vi "TxData_Organization_EVM_EIRP_Max.vi"() -> ()   [LabVIEW 2023, in "ParsingData.lvlib"]
uses:
  <vilib>/Utility/file.llb/Read Delimited Spreadsheet (string).vi
  <vilib>/Utility/file.llb/Read Delimited Spreadsheet (DBL).vi
  ParsingData.lvlib
panel:
  out "Best EVM":T1(array[cluster])
  in  "EIRP_res":dbl=10.0
  in  "EIRP_Max":dbl
  in  "EIRP_Min":dbl=-60.0
  in  "CalPower ¸ÉÀv":dbl=70.0 format="%#_13g"
  in  "Input power_res":dbl=10.0
  in  "Input power_up":dbl
  in  "Input power_low":dbl=-60.0
  in  "File Path":path
  out "Max EVM : Mode             Polarity                     UD att                BFIC COM att           BFIC ele att                SG Power                      EIRP                           EVM":string[](array[string])
  out "EVM to EIRP":cluster{dbl[], "all rows":dbl[]}[](graph)
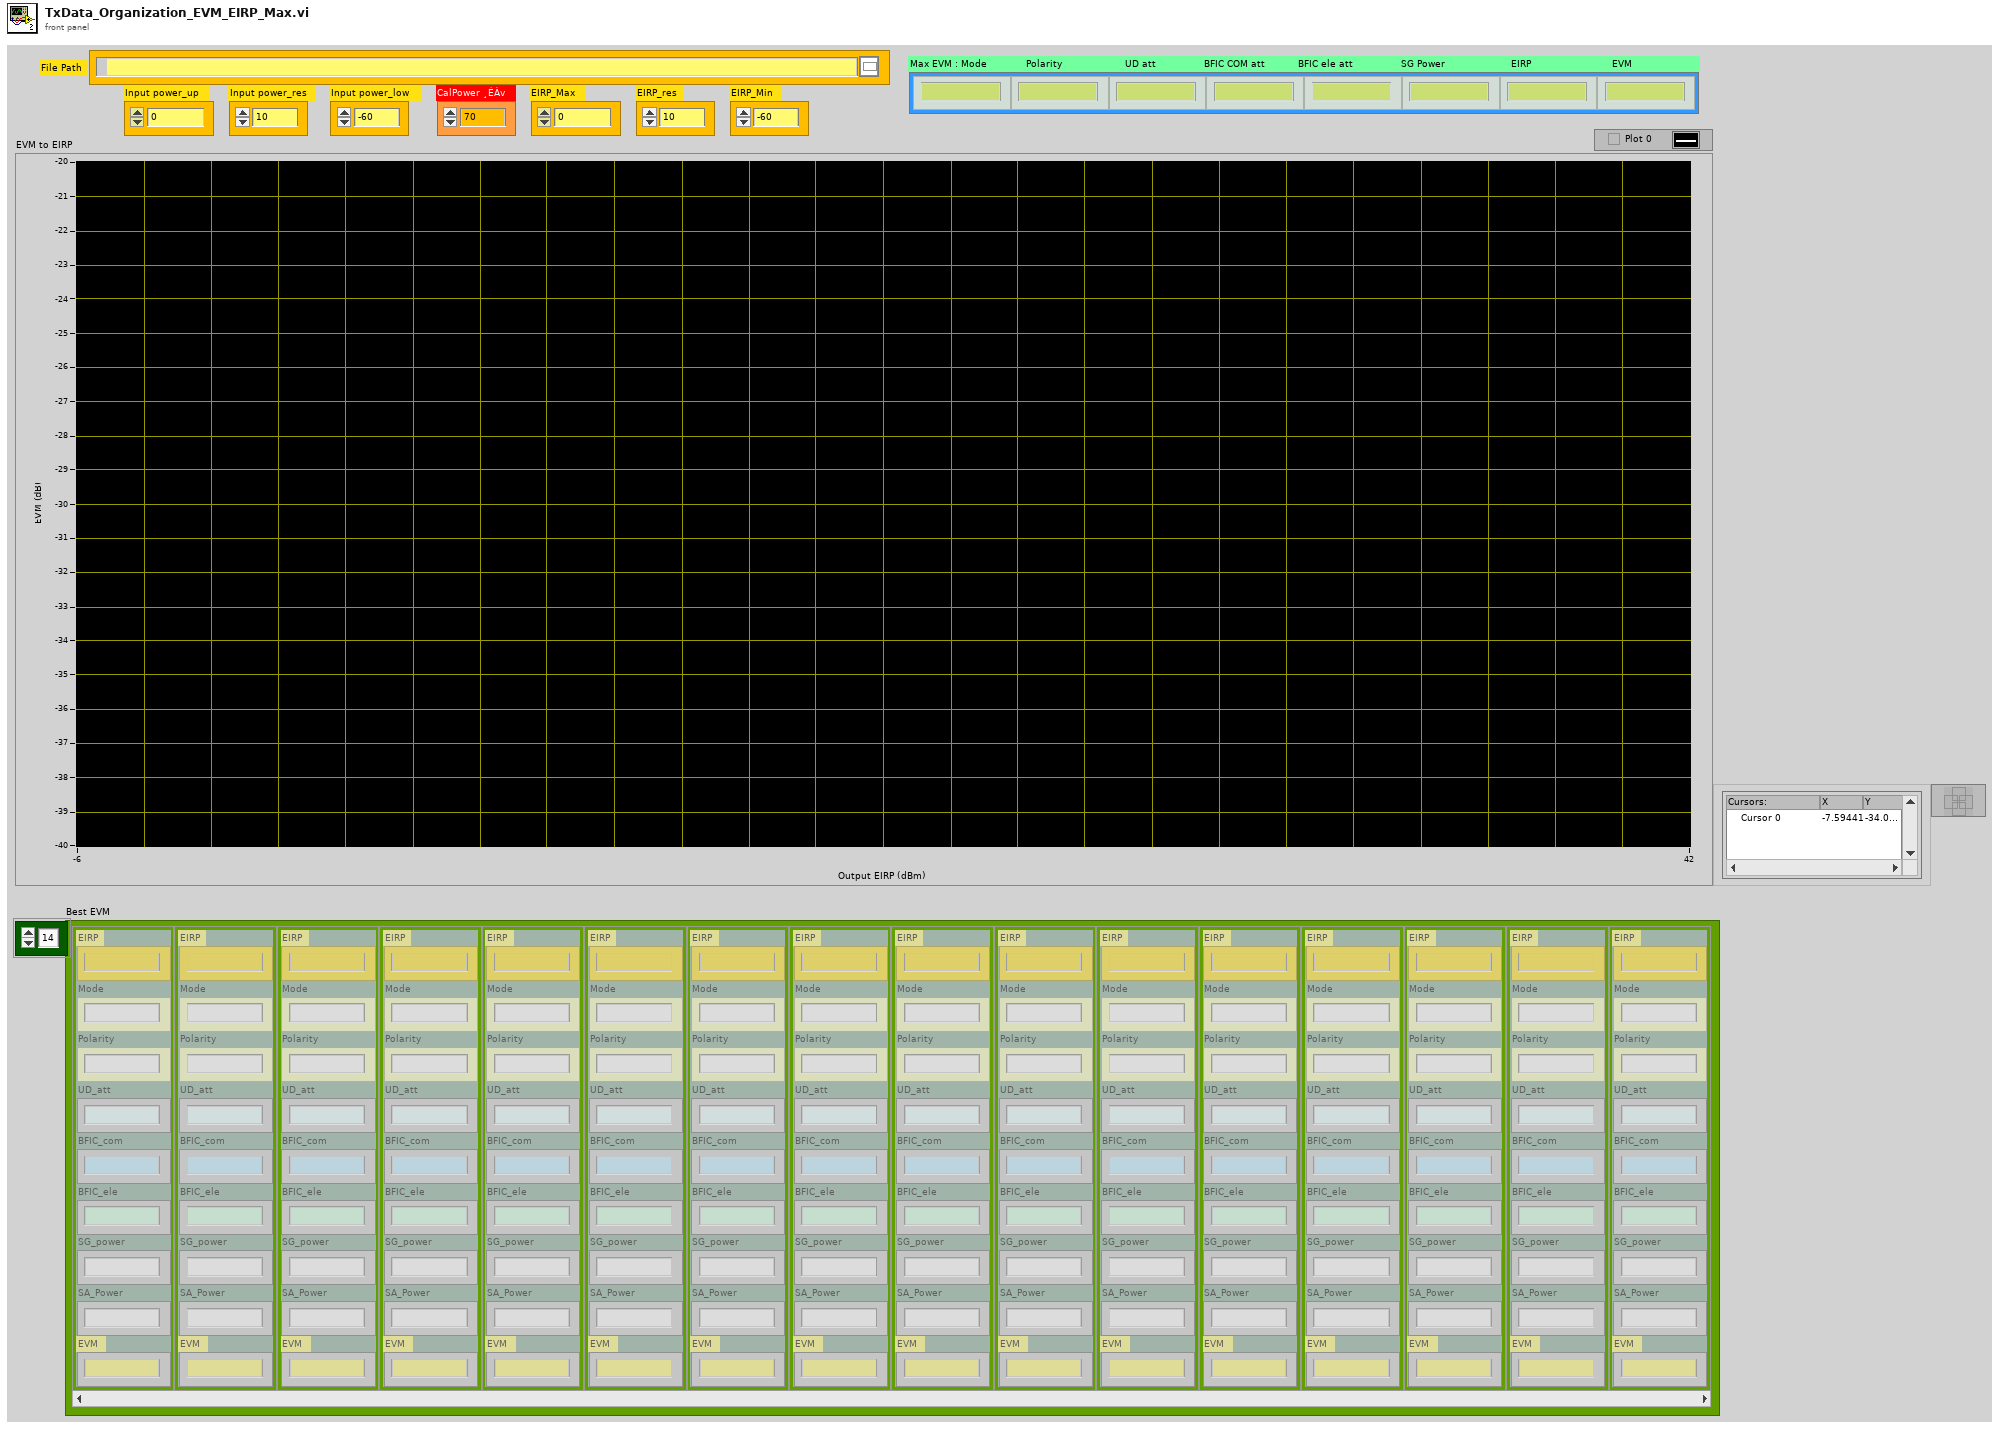
[diagram p1: front panel]
types:
  T1 = cluster{"EIRP":string, "Mode":string, "Polarity":string, "UD_att":string, "BFIC_com":string, "BFIC_ele":string, "SG_power":string, "SA_Power":string, "EVM":string}[]
  T2 = cluster{"[0]":string, "[1]":string, "[2]":string, "[3]":string, "[4]":string, "[5]":string, "[6]":string, "[7]":string, "[8]":string}
  T3 = cluster{"[0]":string, "[1]":string, "[2]":string, "[3]":string, "[4]":string, "[5]":string, "[6]":string, "[7]":string, "[8]":string}[]
  T4 = cluster{"EIRP":string, "Mode":string, "Polarity":string, "UD_att":string, "BFIC_com":string, "BFIC_ele":string, "SG_power":string, "SA_Power":string, "EVM":string}
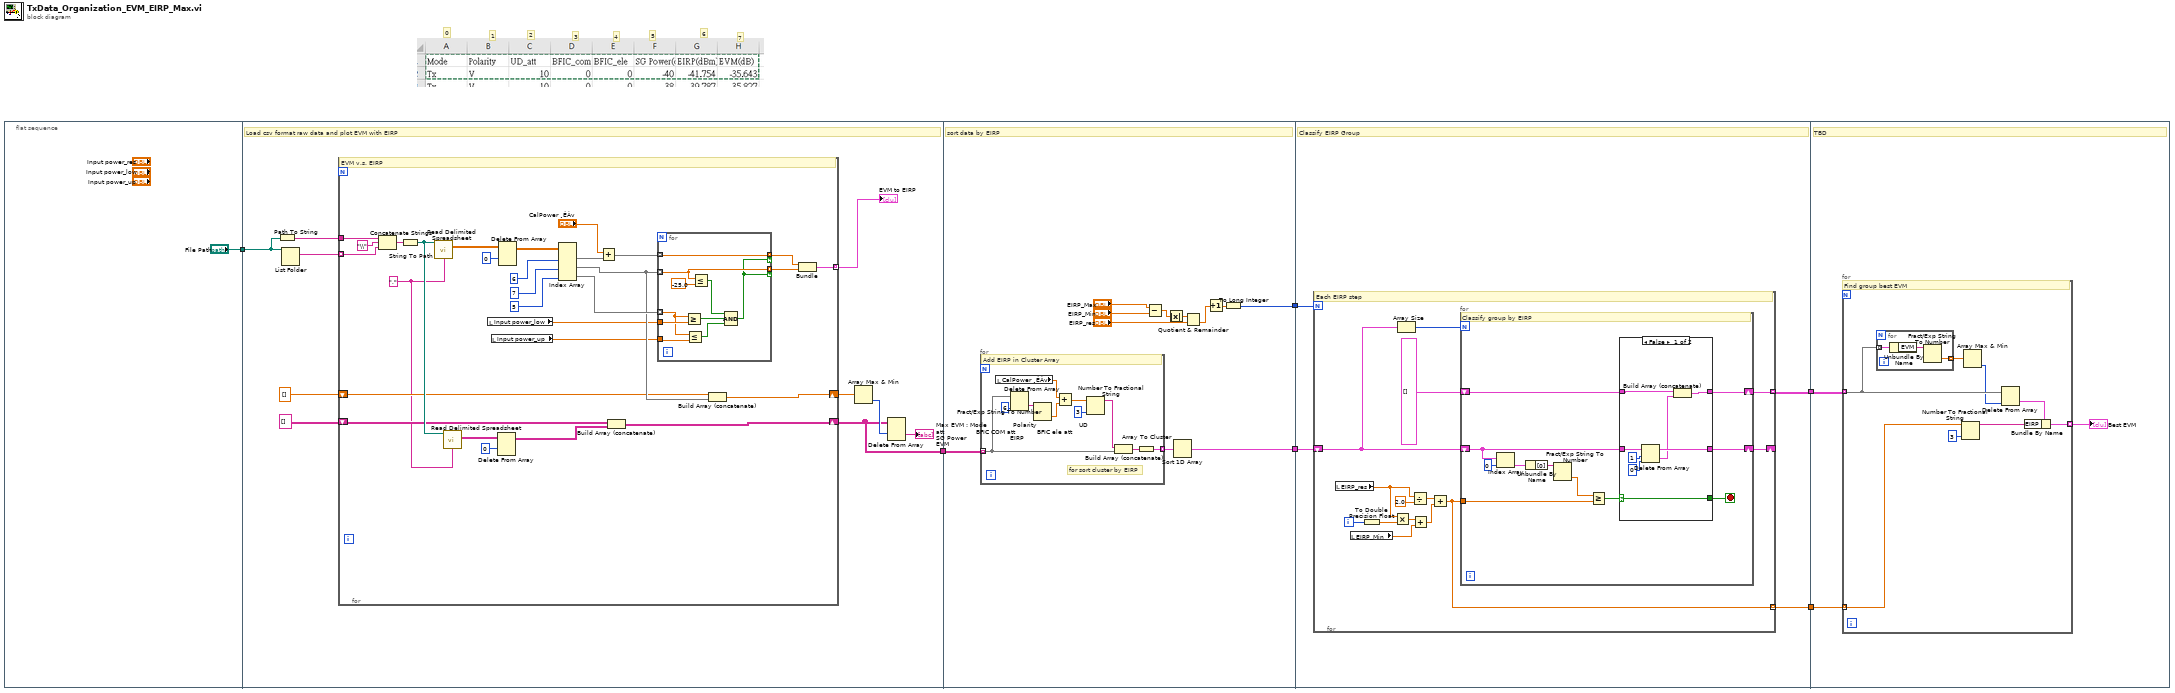
[diagram p0: block diagram]
diagram:
  # "7"
  # "6"
  # "5"
  # "4"
  # "3"
  # "2"
  # "1"
  # "0"
  n1 = flat-sequence {
    tunnel: ["File Path"] -> w5
    tunnel: [w9] -> w6
    tunnel: w5 -> [w11]
    tunnel: w6 -> [w67]
    tunnel: [w57] -> w4
    tunnel: [w61] -> w3
    tunnel: w4 -> [w80]
    tunnel: w3 -> [w81]
    tunnel: [w79] -> w2
    tunnel: [w78] -> w1
    tunnel: w2 -> [w120]
    tunnel: w1 -> [w119]
    frame #0 {
    }
    frame #1 {
      # "Load csv format raw data and plot EVM with EIRP"
      n2 = Path To String(path=w11) -> (string=w16:string)
      n3 = List Folder(path=w11) -> (filenames=w17:string[])  [unwired: 3 in, 3 out]
      n4 = for {
        tunnel: w17 -> [w44] mode=indexing
        tunnel: w16 -> [w46]
        tunnel: [w36] -> w8 mode=indexing
        shift-right: [w20] -> w9
        shift-left: string[][] [] -> [w26]
        shift-right: [w25] -> w14
        shift-left: dbl[] [] -> [w23]
        w22 = "," ("delimiter (\\t)")
        # "EVM v.s. EIRP"
        n5 = Concatenate Strings(w46, "\\" ("string"), w44) -> (w45:string)
        n6 = String To Path(string=w45) -> (path=w28:path)
        n7 = call-poly <vilib>:"Read Delimited Spreadsheet.vi"("file path (dialog if empty)"=w28, "delimiter (\\t)"=w22) -> ("all rows"=w42:dbl[][])  [unwired: 8 in, 5 out]
        n8 = call-poly <vilib>:"Read Delimited Spreadsheet.vi"("file path (dialog if empty)"=w28, "delimiter (\\t)"=w22) -> ("all rows"=w29:string[][])  [unwired: 8 in, 5 out]
        n9 = local read "Input power_low"() -> (w19:dbl)
        n10 = local read "Input power_up"() -> (w18:dbl)
        n11 = Delete From Array(array=w29, index (row)=0 ("disabled index (col)")) -> (array with subset deleted=w27:string[][])  [unwired: 2 in, 1 out]
        n12 = Delete From Array(array=w42, index (row)=0 ("disabled index (col)")) -> (array with subset deleted=w40:dbl[][])  [unwired: 2 in, 1 out]
        n13 = Index Array(array=w40, index (col) #1=6 ("disabled index (col)"), index (col) #2=7 ("index (col)"), index (col) #3=5 ("index (col)")) -> (element #1=w21:dbl[], element #2=w24:dbl[], element #3=w31:dbl[])  [unwired: 3 in]
        n14 = Add(x="CalPower ¸ÉÀv", y=w21) -> (x+y=w35:dbl[])
        n15 = Build Array (concatenate)(w26, w27) -> (w20:string[][])
        n16 = for {
          tunnel: w35 -> [w54] mode=indexing
          tunnel: w24 -> [w55] mode=indexing
          tunnel: [w55] -> w33 mode=indexing if=w47
          tunnel: [w54] -> w34 mode=indexing if=w47
          tunnel: w31 -> [w52] mode=indexing
          tunnel: w19 -> [w53]
          tunnel: w18 -> [w51]
          n17 = Greater Or Equal?(x=w52, y=w53) -> (x >= y?=w49:bool)
          n18 = Less Or Equal?(x=w52, y=w51) -> (x <= y?=w50:bool)
          n19 = Less Or Equal?(x=w55, y=-25.0) -> (x <= y?=w48:bool)
          n20 = Compound Arithmetic op=AND(w48, w49, w50) -> (w47:bool)
        }
        n21 = Build Array (concatenate)(w23, w24) -> (w25:dbl[])
        n22 = Bundle(w34, w33) -> (w36:cluster{dbl[], dbl[]})  [unwired: 1 in]
      }
      "EVM to EIRP" <- w8
      n23 = Array Max & Min(array=w14) -> (min index (indices)=w13:i32)  [unwired: 3 out]
      n24 = Delete From Array(array=w9, index (row)=w13) -> (deleted portion=→"Max EVM : Mode             Polarity                     UD att                BFIC COM att           BFIC ele att                SG Power                      EIRP                           EVM":string[])  [unwired: 2 in, 1 out]
    }
    frame #2 {
      # "sort data by EIRP"
      n25 = for {
        tunnel: w67 -> [w75] mode=indexing
        tunnel: [w77] -> w66 mode=indexing
        # "for sort cluster by EIRP"
        # "Add EIRP in Cluster Array"
        n26 = local read "CalPower ¸ÉÀv"() -> (w70:dbl)
        n27 = Delete From Array(array=w75, index=6) -> (deleted portion=w73:string)  [unwired: 1 in, 1 out]
        n28 = Fract/Exp String To Number(string=w73) -> (number=w71:dbl)  [unwired: 3 in, 1 out]
        n29 = Add(x=w70, y=w71) -> (x+y=w72:dbl)
        n30 = Number To Fractional String(number=w72, precision (6)=i16 3) -> (F-format string=w69:string)  [unwired: 2 in]
        n31 = Build Array (concatenate)(w69, w75) -> (w74:string[])
        n32 = Array To Cluster(array=w74) -> (cluster=w77:T2)
      }
      n33 = Subtract(x="EIRP_Max", y="EIRP_Min") -> (x-y=w65:dbl)
      n34 = Absolute Value(x=w65) -> (abs(x)=w63:dbl)
      n35 = Sort 1D Array(array=w66) -> (sorted array=w57:T3)
      n36 = Quotient & Remainder(x=w63, y="EIRP_res") -> (floor(x/y)=w64:dbl)  [unwired: 1 out]
      n37 = Increment(x=w64) -> (x+1=w62:dbl)
      n38 = To Long Integer(number=w62) -> (32bit integer=w61:i32)
    }
    frame #3 {
      # "Classify EIRP Group"
      n39 = for {
        N: w81 -> [_]
        shift-right: [w86] -> _
        shift-left: w80 -> [w83]
        tunnel: [w87] -> w78 mode=indexing
        tunnel: [w85] -> w79 mode=indexing
        i -> [w91]
        # "Each EIRP step"
        n40 = local read "EIRP_res"() -> (w90:dbl)
        n41 = local read "EIRP_Min"() -> (w88:dbl)
        n42 = To Double Precision Float(number=w91) -> (double precision float=w89:dbl)
        n43 = Multiply(x=w90, y=w89) -> (x*y=w93:dbl)
        n44 = Array Size(array=w83) -> (size(s)=w84:i32)
        n45 = Divide(x=w90, y=2.0) -> (x/y=w94:dbl)
        n46 = Add(x=w93, y=w88) -> (x+y=w95:dbl)
        n47 = Add(x=w94, y=w95) -> (x+y=w87:dbl)
        n48 = for {
          N: w84 -> [_]
          tunnel: w87 -> [w102]
          shift-right: [w96] -> w86
          shift-left: w83 -> [w100]
          shift-right: [w98] -> w85
          shift-left: T1 [] ("reversed array") -> [w99]
          stop <- w97 stop-if-true
          # "Classify group by EIRP"
          n49 = Index Array(array=w100, index=0) -> (element=w106:T2)
          n50 = Unbundle By Name(w106) -> ("[0]"=w103:string)
          n51 = Fract/Exp String To Number(string=w103) -> (number=w104:dbl)  [unwired: 3 in, 1 out]
          n52 = Greater Or Equal?(x=w104, y=w102) -> (x >= y?=w101:bool)
          n53 = case shown="False" w101 {
            selector: w101 -> [w110 w117]
            tunnel: [w110 w117] -> w97
            tunnel: w100 -> [w114 w116]
            tunnel: [w111 w116] -> w96
            tunnel: w99 -> [w109 w115]
            tunnel: [w108 w115] -> w98
            frame False {
              n54 = Delete From Array(array=w114, length=1, index=0) -> (deleted portion=w107:T3, array with subset deleted=w111:T3)
              n55 = Build Array (concatenate)(w109, w107) -> (w108:T3)
            }
            frame True {
            }
          }
        }
      }
    }
    frame #4 {
      # "TBD"
      n56 = for {
        tunnel: w120 -> [w127] mode=indexing
        tunnel: w119 -> [w124] mode=indexing
        tunnel: [w121] -> w118 mode=indexing
        # "Find group best EVM"
        n57 = for {
          tunnel: w127 -> [w131] mode=indexing
          tunnel: [w129] -> w128 mode=indexing
          n58 = Unbundle By Name(w131) -> ("EVM"=w130:string)
          n59 = Fract/Exp String To Number(string=w130) -> (number=w129:dbl)  [unwired: 3 in, 1 out]
        }
        n60 = Number To Fractional String(number=w124, precision (6)=i16 3) -> (F-format string=w123:string)  [unwired: 2 in]
        n61 = Array Max & Min(array=w128) -> (min index (indices)=w126:i32)  [unwired: 3 out]
        n62 = Delete From Array(array=w127, index=w126) -> (deleted portion=w125:T4)  [unwired: 1 in, 1 out]
        n63 = Bundle By Name(cluster=w125, "EIRP"=w123) -> (w121:T4)
      }
      "Best EVM" <- w118
    }
  }
